vi "Get SysCfg Device Info.vi"(6 "Expose System Hardware Reference":bool, 8 "error in":errorcluster, 11 "Refnum in":refnum<k21>) -> (0 "error out":errorcluster, 2 "Network Device":T1 {"Primary Network Adapter"."IP Address Request Mode" items=["Static"=1, "DHCP/Link Local"=2, "Link-Local Only"=4, "DHCP Only"=8]; "Primary Network Adapter"."Adapter Type" items=["Ethernet"=1, "WLAN"=2]; "Primary Network Adapter"."Adapter Mode" items=["Disabled"=1, "TCP/IP Ethernet"=2, "Deterministic"=4, "EtherCAT"=8, "TCP/IP WLAN Connect"=32, "TCP/IP WLAN Create"=64]; "Secondary Network Adapters"."IP Address Request Mode" items=["Static"=1, "DHCP/Link Local"=2, "Link-Local Only"=4, "DHCP Only"=8]; "Secondary Network Adapters"."Adapter Type" items=["Disabled"=1, "TCP/IP Ethernet"=2, "Deterministic"=4, "EtherCAT"=8, "TCP/IP WLAN Connect"=32, "TCP/IP WLAN Create"=64]; "Secondary Network Adapters"."Adapter Mode" items=["Disabled"=1, "TCP/IP Ethernet"=2, "Deterministic"=4, "EtherCAT"=8, "TCP/IP WLAN Connect"=32, "TCP/IP WLAN Create"=64]; "Device Information"."Product ID" format="%.0x"}, 3 "Refnum out":refnum<k21>)   [LabVIEW 2015, in "SMI.lvlib" / "Controller.lvclass"]
uses:
  Controller.lvclass
  Controls/NetworkDevice.ctl
  Controls/DeviceInformation.ctl
  Controls/NetworkAdapterSettings.ctl
  <vilib>/nisyscfg/Find Hardware.vi
  <vilib>/nisyscfg/Close (Resources).vi
  <vilib>/nisyscfg/Close (Filter).vi
  <resource>/objmgr/niflexriosae.rc
  <vilib>/nisyscfg/nisyscfg.lvlib
  <resource>/objmgr/nisysapi.rc
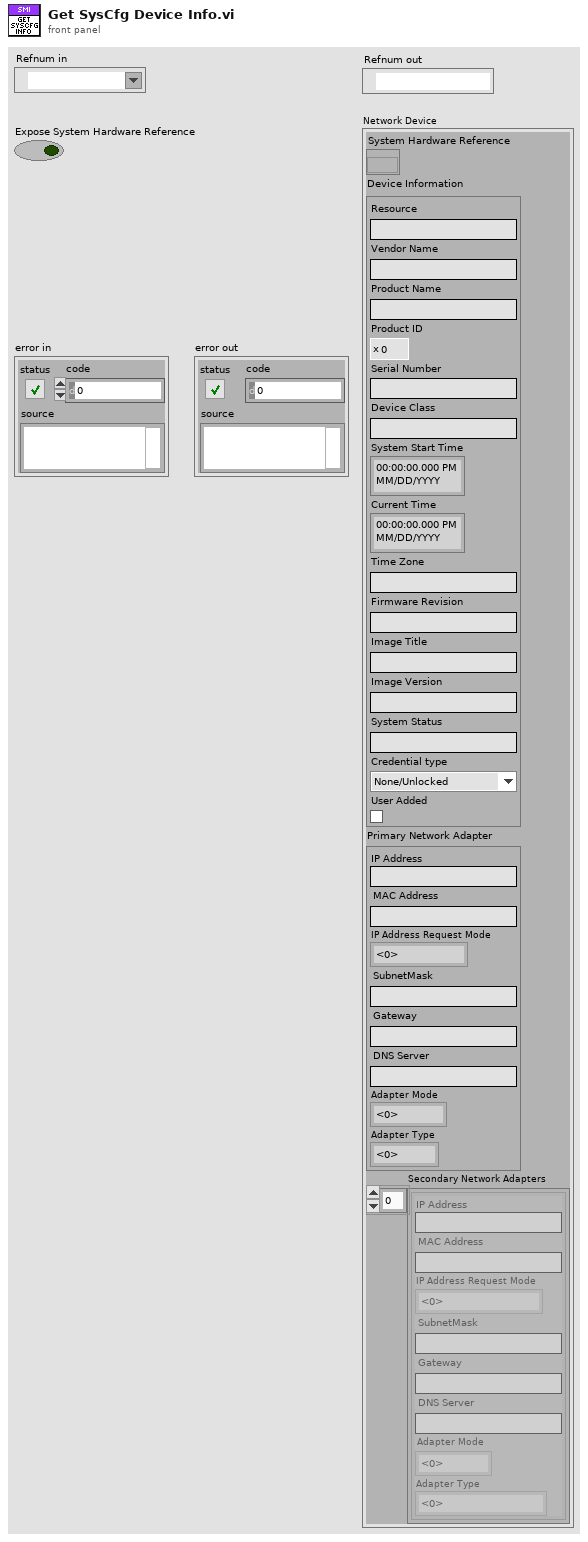
[diagram p1: front panel]
types:
  T1 = typedef "SMI.lvlib/Controller.lvclass/NetworkDevice.ctl" = cluster{"System Hardware Reference":refnum<k20>, "Device Information":T2, "Primary Network Adapter":T3, "Secondary Network Adapters":T3[]}
  T2 = typedef "SMI.lvlib/Controller.lvclass/DeviceInformation.ctl" = cluster{"Resource":string, "Vendor Name":string, "Product Name":string, "Product ID":u32, "Serial Number":string, "Device Class":string, "System Start Time":timestamp, "Current Time":timestamp, "Time Zone":string, "Firmware Revision":string, "Image Title":string, "Image Version":string, "System Status":string, "Credential type":enum16{"None/Unlocked", "FTP Password", "NIAuth Credentials"}, "User Added":bool}
  T3 = typedef "SMI.lvlib/Controller.lvclass/NetworkAdapterSettings.ctl" = cluster{"IP Address":string, "MAC Address":string, "IP Address Request Mode":u32, "SubnetMask":string, "Gateway":string, "DNS Server":string, "Adapter Mode":u32, "Adapter Type":u32}
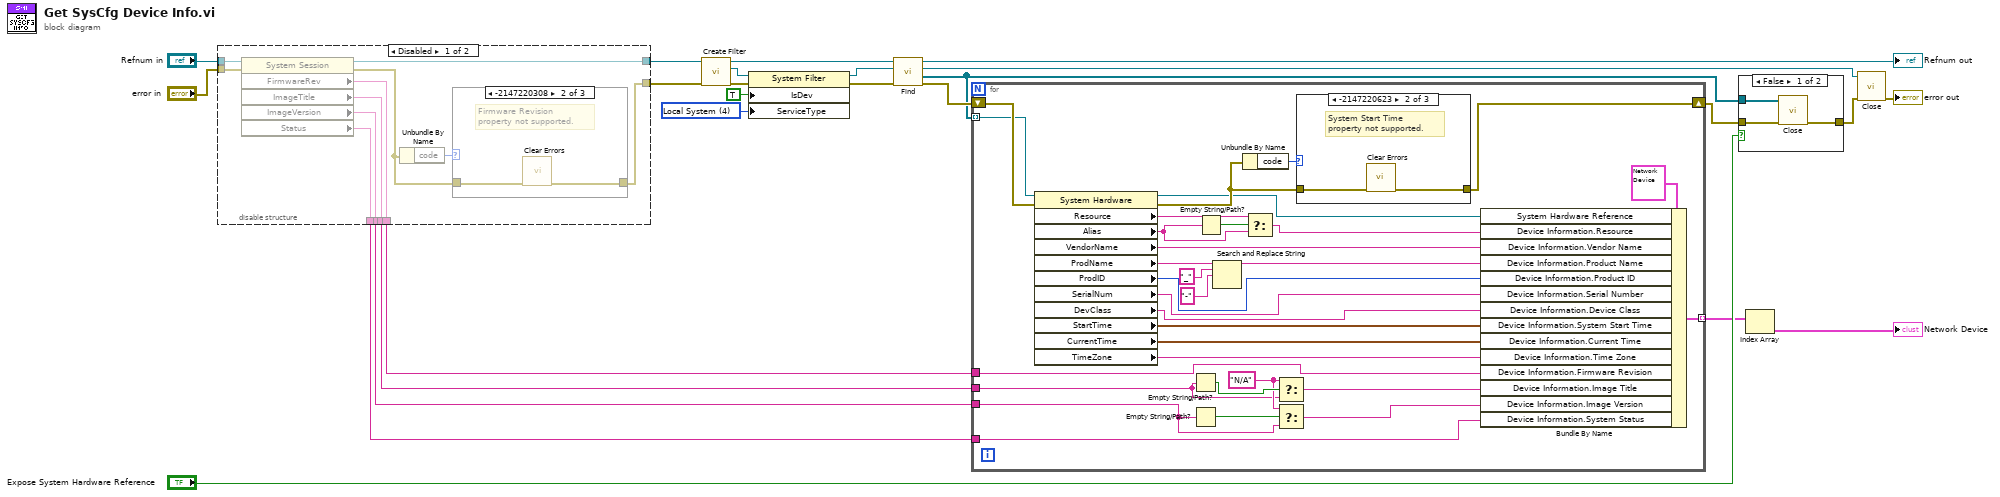
[diagram p0: block diagram]
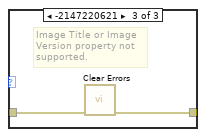
[diagram p3: hidden frame]
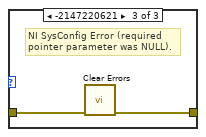
[diagram p7: hidden frame]
diagram:
  w23 = u32 4 items=["NI Network Resource", "NI Real-Time", "NI System Configuration", "NI Web Interface", "Local System", "Local Network Adapter", "Local Time Keeper", "Local Time Reference", "LXI Instrument", "Local FPGA"] ("Service Type")
  n1 = disable-structure shown="Disabled" {
    disable-tunnel: "error in" -> [w35 w41]
    disable-tunnel: "Refnum in" -> [w34 w42]
    disable-tunnel: [w33 _] -> w3
    disable-tunnel: [w32 _] -> w4
    disable-tunnel: [w31 _] -> w5
    disable-tunnel: [w28 _] -> w10
    disable-tunnel: [w27 w41] -> w18
    disable-tunnel: [w26 w42] -> w19
    frame Disabled {
      n2 = property class="System Session"(reference=w34, error in=w35) -> (reference out=w26:refnum<k21>, error out=w30:errorcluster, "FirmwareRev"=w28:string, "ImageTitle"=w31:string, "ImageVersion"=w33:string, "Status"=w32:string)
      n3 = Unbundle By Name(w30) -> ("code"=w29:i32)
      n4 = case shown="-2147220308" w29 {
        tunnel: w30 -> [w36 w38 w40]
        tunnel: [w36 w37 w39] -> w27
        frame Default {
        }
        frame -2147220308 {
          # "Firmware Revision\nproperty not supported."
          n5 = call <vilib>:"Clear Errors.vi"("error in (no error)"=w38) -> ("error out"=w37:errorcluster)  [unwired: 5 in, 1 out]
        }
        frame -2147220621 {
          # "Image Title or Image\nVersion property not \nsupported."
          n6 = call <vilib>:"Clear Errors.vi"("error in (no error)"=w40) -> ("error out"=w39:errorcluster)  [unwired: 5 in, 1 out]
        }
      }
    }
    frame Enabled {
    }
  }
  n7 = call <vilib>:"Create Filter.vi"("error in (no error)"=w18, "Session in"=w19) -> ("error out"=w15:errorcluster, "Filter out"=w16:refnum<k20>, "Session out"=w20:refnum<k21>)  [unwired: 7 in]
  n8 = property class="System Filter"(reference=w16, error in=w15, "IsDev"=TRUE ("Is Device"), "ServiceType"=w23) -> (reference out=w21:refnum<k20>, error out=w17:errorcluster)
  n9 = call-poly <vilib>:"Find.vi"("error in (no error)"=w17, "Filter in"=w21, "Session in"=w20) -> ("error out"=w11:errorcluster, "Resources out"=w8:refnum<k20>[], "Filter out"=w7:refnum<k20>, "Session out"=→"Refnum out":refnum<k21>)  [unwired: 5 in]
  n10 = for {
    tunnel: w3 -> [w46]
    tunnel: w4 -> [w74]
    tunnel: w5 -> [w45]
    tunnel: w8 -> [w51] mode=indexing
    tunnel: [w69] -> w13 mode=indexing
    tunnel: w10 -> [w68]
    shift-right: [w71] -> w9
    shift-left: w11 -> [w67]
    w47 = "N/A"
    n11 = property class="System Hardware"(reference=w51, error in=w67) -> (reference out=w50:refnum<k20>, error out=w73:errorcluster, "Resource"=w64:string, "Alias"=w63:string, "VendorName"=w60:string, "ProdName"=w58:string, "ProdID"=w55:u32, "SerialNum"=w56:string, "DevClass"=w52:string, "StartTime"=w61:timestamp, "CurrentTime"=w65:timestamp, "TimeZone"=w66:string)
    n12 = Empty String/Path?(string/path=w45) -> (empty?=w48:bool)
    n13 = Empty String/Path?(string/path=w46) -> (empty?=w49:bool)
    n14 = Empty String/Path?(string/path=w63) -> (empty?=w62:bool)
    n15 = Search and Replace String(input string=w58, search string="_", replace string="-" ("replace string (\"\")")) -> (result string=w57:string)  [unwired: 5 in, 3 out]
    n16 = Unbundle By Name(w73) -> ("code"=w72:i32)
    n17 = Select(t=w64, s=w62, f=w63) -> (s? t:f=w59:string)
    n18 = Select(t=w47, s=w48, f=w45) -> (s? t:f=w43:string)
    n19 = Select(t=w47, s=w49, f=w46) -> (s? t:f=w44:string)
    n20 = case shown="-2147220623" w72 {
      tunnel: w73 -> [w75 w77 w79]
      tunnel: [w75 w76 w78] -> w71
      frame Default {
      }
      frame -2147220623 {
        # "System Start Time\nproperty not supported."
        n21 = call <vilib>:"Clear Errors.vi"("error in (no error)"=w77) -> ("error out"=w76:errorcluster)  [unwired: 5 in, 1 out]
      }
      frame -2147220621 {
        # "NI SysConfig Error (required\npointer parameter was NULL)."
        n22 = call <vilib>:"Clear Errors.vi"("error in (no error)"=w79) -> ("error out"=w78:errorcluster)  [unwired: 5 in, 1 out]
      }
    }
    n23 = Bundle By Name(cluster=T1 {"System Hardware Reference"=refnum, "Device Information"={"Resource"="", "Vendor Name"="", "Product Name"="", "Product ID"=0, "Serial Number"="", "Device Class"="", "System Start Time"=timestamp(0 s since 1904-01-01), "Current Time"=timestamp(0 s since 1904-01-01), "Time Zone"="", "Firmware Revision"="", "Image Title"="", "Image Version"="", "System Status"="", "Credential type"=enum."None/Unlocked", "User Added"=FALSE}, "Primary Network Adapter"={"IP Address"="", "MAC Address"="", "IP Address Request Mode"=1, "SubnetMask"="", "Gateway"="", "DNS Server"="", "Adapter Mode"=1, "Adapter Type"=1}, "Secondary Network Adapters"=[]} ("Network Device"), "System Hardware Reference"=w50, "Device Information.Resource"=w59, "Device Information.Vendor Name"=w60, "Device Information.Product Name"=w57, "Device Information.Product ID"=w55, "Device Information.Serial Number"=w56, "Device Information.Device Class"=w52, "Device Information.System Start Time"=w61, "Device Information.Current Time"=w65, "Device Information.Time Zone"=w66, "Device Information.Firmware Revision"=w68, "Device Information.Image Title"=w43, "Device Information.Image Version"=w44, "Device Information.System Status"=w74) -> (w69:T1)
  }
  n24 = case shown="False" "Expose System Hardware Reference" {
    tunnel: [w82 w83] -> w6
    tunnel: w8 -> [w81 _]
    tunnel: w9 -> [w80 w83]
    frame False {
      n25 = call-poly <vilib>:"Close.vi"("error in (no error)"=w80, "Resources in"=w81) -> ("error out"=w82:errorcluster)  [unwired: 9 in]
    }
    frame True {
    }
  }
  n26 = Index Array(array=w13) -> (element=→"Network Device":T1)  [unwired: 1 in]
  n27 = call-poly <vilib>:"Close.vi"("error in (no error)"=w6, "Filter in"=w7) -> ("error out"=→"error out":errorcluster)  [unwired: 9 in]
